vi "Maintain Distance.vi"   [LabVIEW 2012, in "Party_Program.exe.lvrbt"]
doc: "This VI is designed to move your Ranger robot so that it maintains a constant distance from a wall or other flat surface. This VI requires an NXT Ultrasonic Sensor on Port 2 and a HITechnic DC Motor Contoller on Port 1. Run this VI and then move your hand or other flat object back and forth in front of the robot. The robot should back away or move closer to the object to maintain a constant distance."
uses:
  Party_Program.exe.lvrbt
  <vilib>/NXT/Block Support/NXT_InputPort.ctl
  <vilib>/NXT/Hardware/Plugins/Tetrix DC Motor/TetrixDCMotorAddress.ctl
  <vilib>/NXT/Dual Mode Library/Display/drawText.vi
  <vilib>/NXT/Dual Mode Library/Sensors/Sonar_cm.vi
  <vilib>/NXT/Dual Mode Library/Waits/Wait_Num.vi
  <vilib>/NXT/NXTIO Xnodes/NXTIONodeSubVIs/TETRIX IO Move DC Motors.vi
  <vilib>/NXT/Subs/LVHSConnector.ctl
  <vilib>/NXT/NXTIO Xnodes/AddressXNode/NXTIOAddress.xnode
  <vilib>/NXT/NXTIO Xnodes/NXTIOXNode/NXTIO.xnode
  <vilib>/NXT/LegoClasses/BrickReference/BrickReference.lvclass
panel:
  # "Press Ctrl + E  (Cmd + E on Mac) to show the block diagram."
types:
  T1 = typedef "LVHSConnector.ctl" = refnum<class "BrickReference.lvclass">
  T2 = typedef "TetrixDCMotorAddress.ctl" = i16
  T3 = cluster{"TetrixDCMotor":T2, "TetrixDCMotor 2":T2}
  T4 = typedef "NXT_InputPort.ctl" = u8
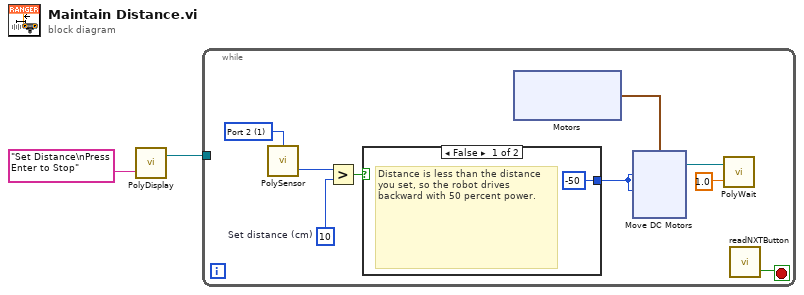
[diagram p0: block diagram]
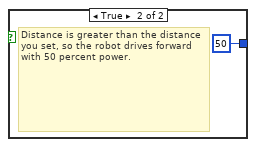
[diagram p2: hidden frame]
diagram:
  n1 = call-poly <vilib>:"PolyDisplay.vi"("Text"="Set Distance\nPress Enter to Stop") -> ("NXT"=w1:T1)  [unwired: 3 in]
  n2 = while {
    tunnel: w1 -> [_]
    stop <- w9 stop-if-true
    w7 = i16 10  # Set distance (cm)
    w10 = T4 1 items=["Port 1", "Port 2", "Port 3", "Port 4"] ("Port (Port 1)")
    n3 = call-poly <vilib>:"PolySensor.vi"("Port (Port 4)"=w10) -> ("Distance (cm)"=w8:i16)  [unwired: 2 in, 1 out]
    n4 = Greater?(x=w8, y=w7) -> (0:w6:bool)
    n5 = case shown="False" w6 {
      tunnel: [i8 -50 ("Power/Speed 1") i8 50 ("Power/Speed 1")] -> w5
      frame False {
        # "Distance is less than the distance you set, so the robot drives backward with 50 percent power."
      }
      frame True {
        # "Distance is greater than the distance you set, so the robot drives forward with 50 percent power."
      }
    }
    n6 = xnode "Motors"() -> ("Motor"=w11:cluster{"TetrixDCMotor":T2, "TetrixDCMotor":T2})
    n7 = xnode "Move DC Motors"("Power/Speed 2"=w5, "Power/Speed 1"=w5, "Motors"=w11) -> ("NXT"=w4:T1)  [unwired: 1 in]
    n8 = call-poly <vilib>:"PolyWait.vi"("Time (1 sec)"=sgl 1.0, "NXT"=w4) -> ()  [unwired: 2 in, 1 out]
    n9 = call <vilib>:"readNXTButton.vi"() -> ("Yes/No"=w9:bool)  [unwired: 3 in, 1 out]
  }
